vi "Backgrounds_171213.vi"(7 "CENTER":enum16{"1", "0"}(ring) caption="Center", 8 "DiameterOfTheMidfield":u8, 9 "DiaMeterOfTheCenter":u8, 10 "MIDFIELD":enum16{"4", "3", "2", "1", "0"}(ring) caption="Midfield", 11 "BORDER":enum16{"8", "6", "5", "4", "3", "2", "1", "0"}(ring) caption="Border") -> (0 "OutputMouseBackground":picture, 1 "NumberedOutput":picture)   [LabVIEW 2016]
uses:
  Globaltracker.vi
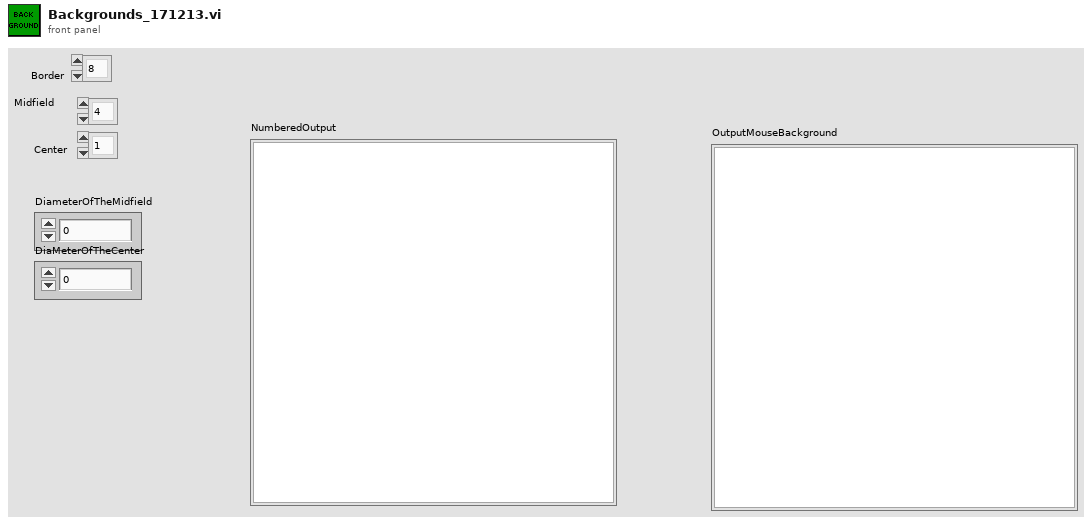
[diagram p1: front panel]
types:
  T1 = cluster{"left":i16, "top":i16, "right":i16, "bottom":i16}
  T2 = cluster{"Width":u16, "Style":enum32{"Solid", "Dash", "Dot", "DashDot", "DashDotDot"}}
  T3 = typedef "imagedata.ctl" = cluster{"image type":i32, "image depth":i32, "image":u8[], "mask":u8[], "colors":u32[], "Rectangle":cluster{"left":i16, "top":i16, "right":i16, "bottom":i16}}
  T4 = cluster{"horizontal":enum16{"left", "center", "right"}, "vertical":enum16{"top", "center", "bottom"}}
  T5 = cluster{"Font Name:":string, "Size":i16, "Strikeout?":bool, "Italic?":bool, "Underline?":bool, "Outline?":bool, "Shadow?":bool, "Bold?":bool}
  T6 = enum16{"User-specified Font", "Application Font", "System Font", "Dialog Font"}
  T7 = cluster{"Font Name:":string, i16, "Strikeout?":bool, "Italic?":bool, "Underline?":bool, "Outline?":bool, "Shadow?":bool, "Bold?":bool}
  T8 = cluster{"image type":i32, "image depth":i32, "image":u8[], "mask":u8[], "colors":u32[], cluster{i32, i32, i32, i32}}
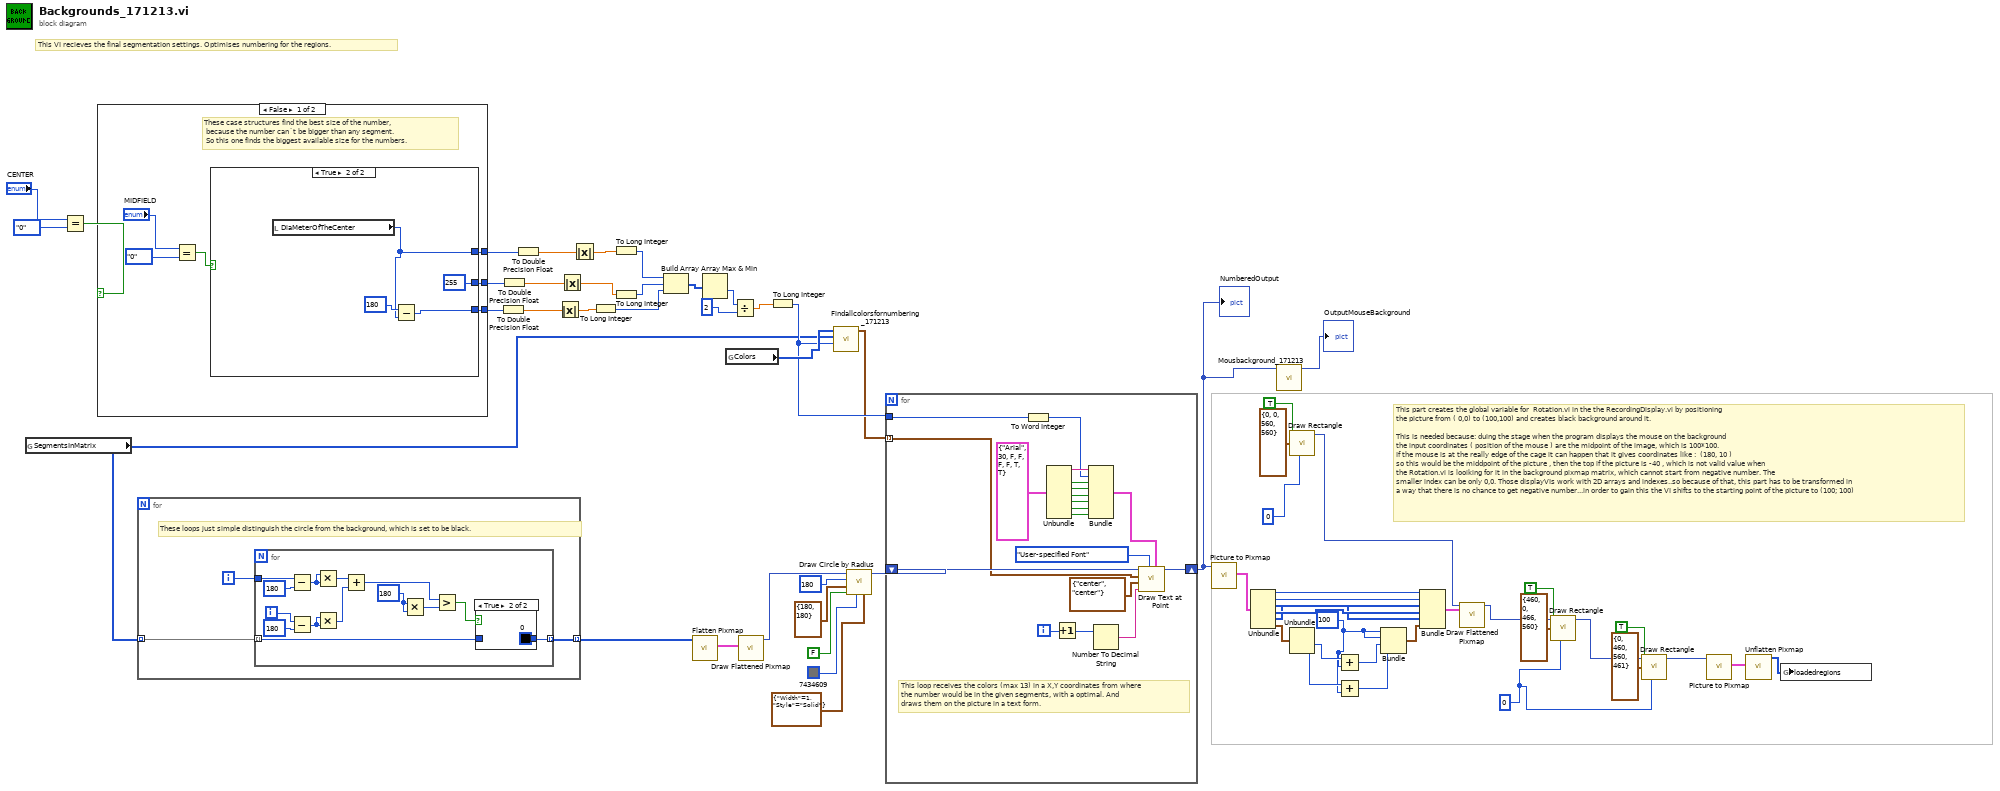
[diagram p0: block diagram]
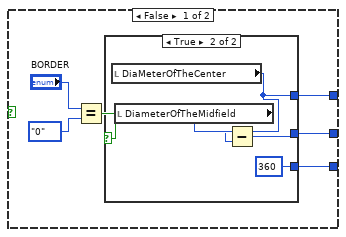
[diagram p2: hidden frame]
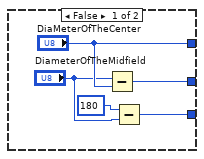
[diagram p3: hidden frame]
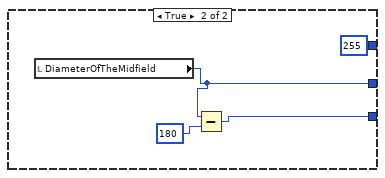
[diagram p4: hidden frame]
diagram:
  w11 = 0
  w29 = 100
  # "This part creates the global variable for  Rotation.vi in the the RecordingDisplay.vi by positioning \nthe picture from ( 0,0) to (100,100) and creates black background around it.\n\nThis is needed because: duing the stage when the program displays the mouse on the background\nthe input coordinates ( position of the mouse ) are the midpoint of the image, which is 100*100. \nIf the mouse is at the really edge of the cage it can happen that it gives coordinates like :  (180, 10 )\nso this would be the middpoint of the picture , then the top if the picture is -40 , which is not valid value when \nthe Rotation.vi is looiking for it in the background pixmap matrix, which cannot start from negative number. The \nsmaller index can be only 0,0. Those displayVIs work with 2D arrays and indexes..so because of that, this part has to be transformed in \na way that there is no chance to get negative number...in order to gain this the VI shifts to the starting point of the picture to (100; 100)"
  # "This VI recieves the final segmentation settings. Optimises numbering for the regions."
  n1 = global read "Globaltracker.vi" "SegmentsInMatrix"() -> (w36:u32[][])
  n2 = Equal?(x="CENTER", y=enum16{"1", "0"}."0") -> (x = y?=w51:bool)
  n3 = case shown="False" w51 {
    tunnel: [w67 u8 255 ("Diameter of the center")] -> w45
    tunnel: [w66 w89] -> w48
    tunnel: [w65 w88] -> w47
    frame False {
      # "These case structures find the best size of the number,\n because the number can´t be bigger than any segment.\n So this one finds the biggest available size for the numbers."
      n4 = Equal?(x="MIDFIELD", y=enum16{"4", "3", "2", "1", "0"}."0") -> (x = y?=w68:bool)
      n5 = case shown="True" w68 {
        tunnel: [w73 w85] -> w67
        tunnel: [w72 u8 255] -> w66
        tunnel: [w71 w84] -> w65
        frame False {
          n6 = Equal?(x="BORDER", y=enum16{"8", "6", "5", "4", "3", "2", "1", "0"}."0") -> (x = y?=w74:bool)
          n7 = case shown="True" w74 {
            tunnel: ["DiaMeterOfTheCenter" w82] -> w73
            tunnel: [w78 w81] -> w72
            tunnel: [w75 360] -> w71
            frame False {
              n8 = Subtract(x="DiameterOfTheMidfield", y="DiaMeterOfTheCenter") -> (x-y=w78:u8)
              n9 = Subtract(x=180, y="DiameterOfTheMidfield") -> (x-y=w75:i32)
            }
            frame True {
              n10 = local read "DiaMeterOfTheCenter"() -> (w82:u8)
              n11 = local read "DiameterOfTheMidfield"() -> (w83:u8)
              n12 = Subtract(x=w83, y=w82) -> (x-y=w81:u8)
            }
          }
        }
        frame True {
          n13 = local read "DiaMeterOfTheCenter"() -> (w85:u8)
          n14 = Subtract(x=180, y=w85) -> (x-y=w84:i32)
        }
      }
    }
    frame True {
      n15 = local read "DiameterOfTheMidfield"() -> (w89:u8)
      n16 = Subtract(x=w89, y=180) -> (x-y=w88:i32)
    }
  }
  n17 = for {
    tunnel: w36 -> [w94] mode=indexing
    tunnel: [w92] -> w55 mode=indexing
    i -> [w93]
    # "These loops just simple distinguish the circle from the background, which is set to be black."
    n18 = for {
      tunnel: w94 -> [w96] mode=indexing
      tunnel: w93 -> [w100]
      tunnel: [w95] -> w92 mode=indexing
      i -> [w99]
      w98 = 180 ("y")
      n19 = Subtract(x=w100, y=180) -> (x-y=w103:i32)
      n20 = Subtract(x=w99, y=180) -> (x-y=w104:i32)
      n21 = Multiply(x=w103, y=w103) -> (x*y=w106:i32)
      n22 = Multiply(x=w104, y=w104) -> (x*y=w105:i32)
      n23 = Add(x=w106, y=w105) -> (x+y=w108:i32)
      n24 = Multiply(x=w98, y=w98) -> (x*y=w107:i32)
      n25 = Greater?(x=w108, y=w107) -> (0:w97:bool)
      n26 = case shown="True" w97 {
        tunnel: w96 -> [w109 _]
        tunnel: [w109 u32 0 ("color(black)")] -> w95
        frame False {
        }
        frame True {
        }
      }
    }
  }
  n27 = To Double Precision Float(number=w47) -> (double precision float=w42:dbl)
  n28 = To Double Precision Float(number=w48) -> (double precision float=w43:dbl)
  n29 = To Double Precision Float(number=w45) -> (double precision float=w44:dbl)
  n30 = Absolute Value(x=w42) -> (abs(x)=w39:dbl)
  n31 = Absolute Value(x=w43) -> (abs(x)=w40:dbl)
  n32 = Absolute Value(x=w44) -> (abs(x)=w41:dbl)
  n33 = To Long Integer(number=w39) -> (32bit integer=w46:i32)
  n34 = To Long Integer(number=w41) -> (32bit integer=w50:i32)
  n35 = To Long Integer(number=w40) -> (32bit integer=w49:i32)
  n36 = Build Array(w50, w49, w46) -> (w3:i32[])
  n37 = call <vilib>:"Flatten Pixmap.vi"("24-bit pixmap"=w55) -> ("image data"=w62:T3)  [unwired: 10 in]
  n38 = Array Max & Min(array=w3) -> (min value=w54:i32)  [unwired: 3 out]
  n39 = global read "Globaltracker.vi" "Colors"() -> (w38:u32[])
  n40 = Divide(x=w54, y=2) -> (x/y=w52:dbl)
  n41 = call <vilib>:"Draw Flattened Pixmap.vi"("image data"=w62) -> ("new picture"=w60:picture)  [unwired: 8 in]
  n42 = To Long Integer(number=w52) -> (32bit integer=w37:i32)
  n43 = call "Findallcolorsfornumbering_171213.vi"("Size"=w37, "Input2Darray(SegmentedCircle)"=w36, "Colors"=w38) -> ("Numbering coordinates"=w10:cluster{i32, i32}[])  [unwired: 8 in]
  n44 = call <vilib>:"Draw Circle by Radius.vi"("pen"=T2 {"Width"=1, "Style"=enum."Solid"}, "color(black)"=u32 7434609, "fill?(F)"=FALSE, "pixel center"=cluster{"horizontal":i16, "vertical":i16} {"horizontal"=180, "vertical"=180}, "radius"=i16 180, "picture"=w60) -> ("new picture"=w53:picture)  [unwired: 5 in]
  n45 = for {
    shift-right: [w126] -> w1
    shift-left: w53 -> [w129]
    tunnel: w37 -> [w111]
    tunnel: w10 -> [w114] mode=indexing
    i -> [w113]
    # "This loop receives the colors (max 13) in a X,Y coordinates from where\nthe number would be in the given segments, with a optimal. And\ndraws them on the picture in a text form."
    n46 = To Word Integer(number=w111) -> (16bit integer=w116:i16)
    n47 = Unbundle(T5 {"Font Name:"="Arial", "Size"=30, "Strikeout?"=FALSE, "Italic?"=FALSE, "Underline?"=FALSE, "Outline?"=FALSE, "Shadow?"=TRUE, "Bold?"=TRUE} ("[user-specified font]")) -> ("Font Name:"=w123:string, "Strikeout?"=w117:bool, "Italic?"=w118:bool, "Underline?"=w119:bool, "Outline?"=w120:bool, "Shadow?"=w121:bool, "Bold?"=w122:bool)  [unwired: 1 out]
    n48 = Increment(x=w113) -> (x+1=w112:i32)
    n49 = Bundle("Font Name:"=w123, w116, "Strikeout?"=w117, "Italic?"=w118, "Underline?"=w119, "Outline?"=w120, "Shadow?"=w121, "Bold?"=w122) -> (w115:T7)  [unwired: 1 in]
    n50 = Number To Decimal String(number=w112) -> (decimal integer string=w125:string)  [unwired: 1 in]
    n51 = call <vilib>:"Draw Text at Point.vi"("[user-specified font]"=w115, "desired font(Application)"=T6."User-specified Font", "text"=w125, "alignment(left, top)"=T4 {"horizontal"=enum."center", "vertical"=enum."center"}, "origin"=w114, "picture"=w129) -> ("new picture"=w126:picture)  [unwired: 4 in, 1 out]
  }
  "NumberedOutput" <- w1
  n52 = call <vilib>:"Picture to Pixmap.vi"("picture"=w1) -> ("image data"=w33:T3)  [unwired: 9 in, 1 out]
  n53 = Unbundle(w33) -> ("image type"=w26:i32, "image depth"=w25:i32, "image"=w24:u8[], "mask"=w23:u8[], "colors"=w22:u32[], "Rectangle"=w32:T1)
  n54 = call "Mousbackground_171213.vi"("input"=w1) -> ("output-background"=→"OutputMouseBackground":picture)  [unwired: 10 in]
  n55 = call <vilib>:"Draw Rectangle.vi"("rect"=T1 {"left"=0, "top"=0, "right"=560, "bottom"=560}, "fill?(F)"=TRUE, "color(black)"=0) -> ("new picture"=w19:picture)  [unwired: 6 in]
  n56 = Unbundle(w32) -> ("right"=w31:i16, "bottom"=w30:i16)  [unwired: 2 out]
  n57 = Add(x=w31, y=w29) -> (x+y=w28:i32)
  n58 = Add(x=w30, y=w29) -> (x+y=w27:i32)
  n59 = Bundle(w29, w29, w28, w27) -> (w21:cluster{i32, i32, i32, i32})  [unwired: 1 in]
  n60 = Bundle("image type"=w26, "image depth"=w25, "image"=w24, "mask"=w23, "colors"=w22, w21) -> (w20:T8)  [unwired: 1 in]
  n61 = call <vilib>:"Draw Flattened Pixmap.vi"("image data"=w20, "picture"=w19) -> ("new picture"=w16:picture)  [unwired: 7 in]
  n62 = call <vilib>:"Draw Rectangle.vi"("picture"=w16, "rect"=T1 {"left"=460, "top"=0, "right"=466, "bottom"=560}, "fill?(F)"=TRUE, "color(black)"=w11) -> ("new picture"=w12:picture)  [unwired: 5 in]
  n63 = call <vilib>:"Draw Rectangle.vi"("picture"=w12, "rect"=T1 {"left"=0, "top"=460, "right"=560, "bottom"=461}, "fill?(F)"=TRUE, "color(black)"=w11) -> ("new picture"=w7:picture)  [unwired: 5 in]
  n64 = call <vilib>:"Picture to Pixmap.vi"("picture"=w7) -> ("image data"=w9:T3)  [unwired: 9 in, 1 out]
  n65 = call <vilib>:"Unflatten Pixmap.vi"("image data"=w9) -> ("24-bit pixmap"=w8:u32[][])  [unwired: 4 in, 6 out]
  n66 = global write "Globaltracker.vi" "loadedregions"(w8) -> ()
